vi "Clear Chart Data.vi"(8 "error in (no error)":errorcluster, 11 "WaveformChart in":refnum<vi>) -> (0 "error out":errorcluster)   [LabVIEW 2014, in "Chart Module.lvlib"]
uses:
  Chart Module.lvlib
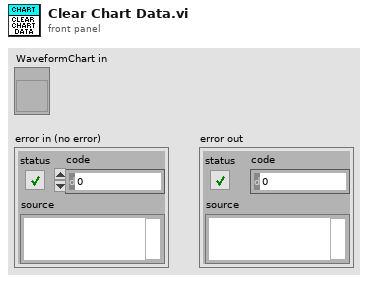
[diagram p1: front panel]
types:
  T1 = cluster{"Value":dbl, "HighLim":dbl, "LowLim":dbl}[]
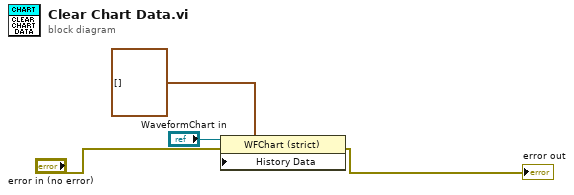
[diagram p0: block diagram]
diagram:
  n1 = property on="Property Node" class="WFChart (strict)"(reference="WaveformChart in", error in="error in (no error)", "History Data"=T1 []) -> (error out=→"error out":errorcluster)  [unwired: 1 out]
